vi "Update Buttons.vi"(8 "error in (no error)":errorcluster, 11 "GripsMaster in":refnum<class "GripsMaster.lvclass">) -> (0 "error out":errorcluster, 3 "GripsMaster out":refnum<class "GripsMaster.lvclass">)   [LabVIEW 2011, in "GripsMaster.lvclass"]
uses:
  GripsMaster.lvclass
  GripsMaster.lvclass/GripsMaster.ctl
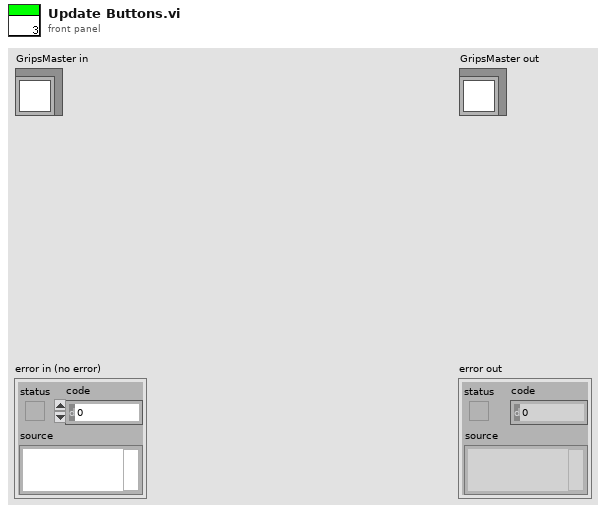
[diagram p1: front panel]
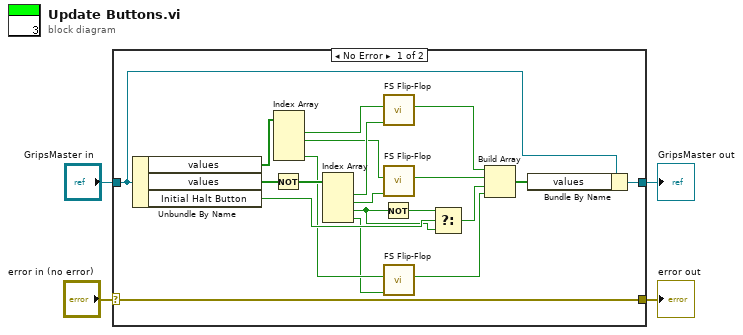
[diagram p0: block diagram]
diagram:
  n1 = case shown="No Error" "error in (no error)" {
    selector: "error in (no error)" -> [w24 w26]
    tunnel: [w24 w26] -> w3
    tunnel: [w22 w25] -> w1
    tunnel: "GripsMaster in" -> [w21 w25]
    frame No Error {
      n2 = Unbundle By Name(w21) -> ("values"=w13:bool[], "values"=w23:bool[], "Initial Halt Button"=w16:bool)
      n3 = Not(x=w23) -> (.not. x?=w19:bool[])
      n4 = Index Array(array=w13) -> (element #1=w12:bool, element #2=w9:bool, element #4=w6:bool)  [unwired: 4 in, 1 out]
      n5 = Index Array(array=w19) -> (element #1=w14:bool, element #2=w8:bool, element #3=w15:bool, element #4=w5:bool)  [unwired: 4 in]
      n6 = Not(x=w15) -> (.not. x?=w20:bool)
      n7 = call "FS Flip-Flop.vi"("Button Value"=w14, "Current State"=w12) -> ("result"=w11:bool)  [unwired: 9 in]
      n8 = call "FS Flip-Flop.vi"("Button Value"=w8, "Current State"=w9) -> ("result"=w10:bool)  [unwired: 9 in]
      n9 = call "FS Flip-Flop.vi"("Button Value"=w5, "Current State"=w6) -> ("result"=w7:bool)  [unwired: 9 in]
      n10 = Select(t=w20, s=w16, f=w15) -> (s? t:f=w18:bool)
      n11 = Build Array(w11, w10, w18, w7) -> (w17:bool[])
      n12 = Bundle By Name(cluster=w21, "values"=w17) -> (w22:refnum<class "GripsMaster.lvclass">)
    }
    frame Error {
    }
  }
  "error out" <- w3
  "GripsMaster out" <- w1
